vi "Exemple_Impute_IterativeImputer.vi"() -> ()   [LabVIEW 2020]
uses:
  Objet/6 - Datasets Transformation/6.4 - Imputation of missing values/IterativeImputer/IterativeImputer.lvclass
panel:
  in  "IterativeImputer":T1={"estimator"="None", "missing_values"="nan", "sample_posterior"=FALSE, "max_iter"=10, "tol"=0.001, "n_nearest_features"=-1, "initial_strategy"="mean", "imputation_order"="ascending", "skip_complete"=FALSE, "min_value"=["None"], "max_value"=["None"], "verbose"=0, "random_state"=-1, "add_indicator"=FALSE} {"random_state" min=-1; "n_nearest_features" min=-1}
  out "Data":T2
  out "error out":errorcluster caption="sortie d'erreur"
  in  "y":string[][](array[string])
  in  "X":string[][](array[string])=[["nan", "2", "3"], ["4", "nan", "6"], ["10", "nan", "9"]]
  in  "error in":errorcluster caption="entrée d'erreur"
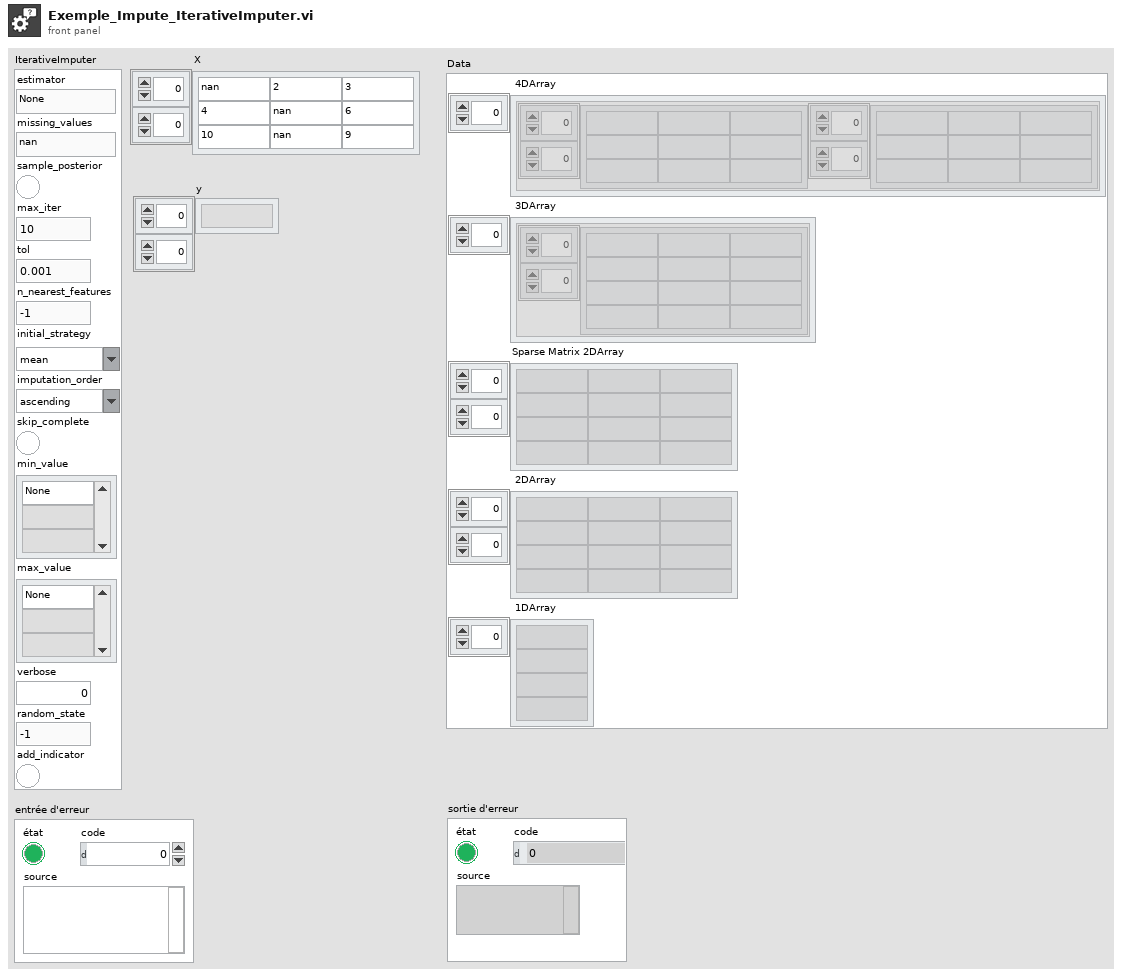
[diagram p1: front panel]
types:
  T1 = cluster{"estimator":string, "missing_values":string, "sample_posterior":bool, "max_iter":i32, "tol":dbl, "n_nearest_features":i32, "initial_strategy":string, "imputation_order":string, "skip_complete":bool, "min_value":string[], "max_value":string[], "verbose":i32, "random_state":i32, "add_indicator":bool}
  T2 = cluster{" 4DArray":cluster{"1":string[][], "2":string[][]}[], " 3DArray":cluster{"Tableau":string[][]}[], "Sparse Matrix 2DArray":string[][], " 2DArray":string[][], " 1DArray":string[]}
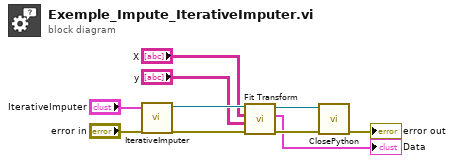
[diagram p0: block diagram]
diagram:
  n1 = call "IterativeImputer.vi"("error in"="error in", "IterativeImputer"="IterativeImputer") -> ("error out"=w9:errorcluster, "IterativeImputer.lvclass"=w5:refnum<class "IterativeImputer.lvclass">)  [unwired: 8 in]
  n2 = call-dynamic "Fit Transform.vi"("error in (no error)"=w9, "y"="y", "X"="X", "IterativeImputer.lvclass"=w5) -> ("error out"=w6:errorcluster, "Data"=→"Data":T2, "IterativeImputer.lvclass"=w7:refnum<class "IterativeImputer.lvclass">)  [unwired: 5 in]
  n3 = call-dynamic "ClosePython.vi"("error in (no error)"=w6, "Scikit-learn en entrée"=w7) -> ("error out"=→"error out":errorcluster)  [unwired: 8 in, 1 out]
